vi "CheckFileWriteStatus-v1.vi"(5 "WriteDataButtonVal":bool, 7 "WritePrevVal":bool, 9 "Refnum in":refnum<k34>, 10 "Base filename":string, 11 "File path":path) -> (0 "File Name":string, 1 "Refnum out":refnum<k34>, 3 "WriteCurrentVal":bool)   [LabVIEW 2018]
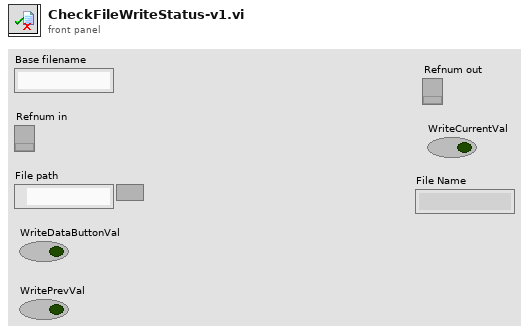
[diagram p1: front panel]
types:
  T1 = enum16{"open", "open or create", "create or replace", "create", "open (read-only)"}
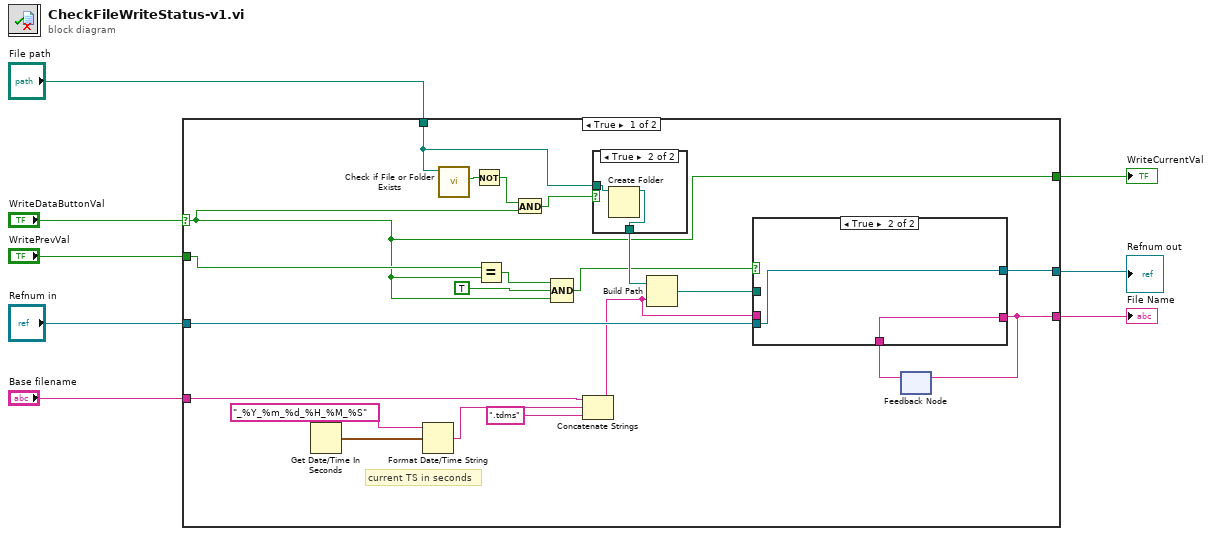
[diagram p0: block diagram]
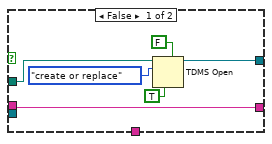
[diagram p3: hidden frame]
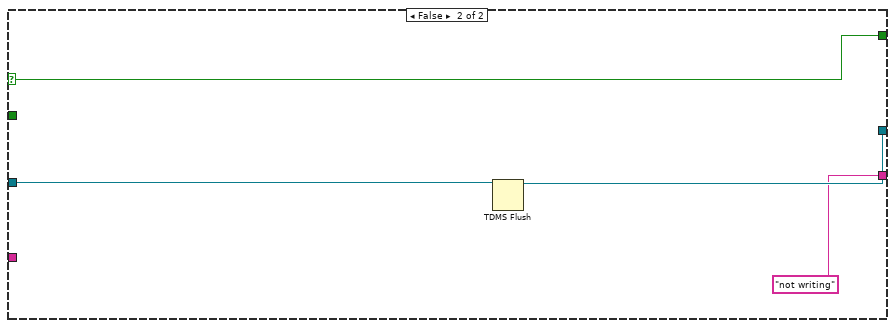
[diagram p4: hidden frame]
diagram:
  n1 = case shown="True" "WriteDataButtonVal" {
    selector: "WriteDataButtonVal" -> [w14 w42]
    tunnel: [w26 w43] -> w7
    tunnel: "Refnum in" -> [w24 w44]
    tunnel: [w14 w42] -> w6
    tunnel: "WritePrevVal" -> [w18 _]
    tunnel: "File path" -> [w13 _]
    tunnel: "Base filename" -> [w12 _]
    tunnel: [w10 "not writing"] -> w1
    frame True {
      # "current TS in seconds"
      n2 = Get Date/Time In Seconds() -> (seconds since 1Jan1904=w28:timestamp)
      n3 = Format Date/Time String(time format string (%c)="_%Y_%m_%d_%H_%M_%S", seconds (now)=w28) -> (date/time string=w29:string)  [unwired: 1 in]
      n4 = call <vilib>:"Check if File or Folder Exists.vi"("path"=w13) -> ("file or folder exists?"=w22:bool)  [unwired: 8 in, 2 out]
      n5 = Not(x=w22) -> (.not. x?=w20:bool)
      n6 = Equal?(x=w18, y=w14) -> (x = y?=w17:bool)
      n7 = And(x=w20, y=w14) -> (x .and. y?=w21:bool)
      n8 = Compound Arithmetic op=AND(w17, TRUE ("y"), w14) -> (w15:bool)
      n9 = Concatenate Strings(w12, w29, ".tdms" ("string")) -> (w11:string)
      n10 = case shown="True" w21 {
        tunnel: w13 -> [w30 w32]
        tunnel: [w30 w31] -> w23
        frame False {
        }
        frame True {
          n11 = Create Folder(path (use dialog)=w32) -> (created path=w31:path)  [unwired: 2 in, 2 out]
        }
      }
      n12 = Build Path(base path=w23, name or relative path=w11) -> (appended path=w19:path)
      n13 = feedback #1() -> (w9:string)  [unwired: 1 in]
      n14 = case shown="True" w15 {
        tunnel: [w35 w40] -> w26
        tunnel: w19 -> [w34 _]
        tunnel: w24 -> [_ w40]
        tunnel: [w33 w39] -> w10
        tunnel: w11 -> [w33 _]
        tunnel: w9 -> [_ w39]
        frame False {
          n15 = TDMS Open(5:FALSE ("create index file? (T)"), 6:TRUE ("disable buffering (T)"), 10:T1."create or replace" ("operation"), 11:w34) -> (3:w35:refnum<k34>)  [unwired: 3 in, 1 out]
        }
        frame True {
        }
      }
      n16 = feedback-in #1(w10) -> ()
    }
    frame False {
      n17 = TDMS Flush(7:w44) -> (3:w43:refnum<k34>)  [unwired: 1 in, 1 out]
    }
  }
  "Refnum out" <- w7
  "WriteCurrentVal" <- w6
  "File Name" <- w1
